vi "Radau5_Timestep Check.vi"(0 "time step":dbl, 5 "Initial time step":dbl, 7 "Max time step":dbl, 9 "Min time step":dbl, 11 "error in (no error)":errorcluster) -> (15 "error out":errorcluster)   [LabVIEW 2020, in "NI_DAE.lvlib"]
uses:
  <vilib>/gmath/NI_DAE.lvlib
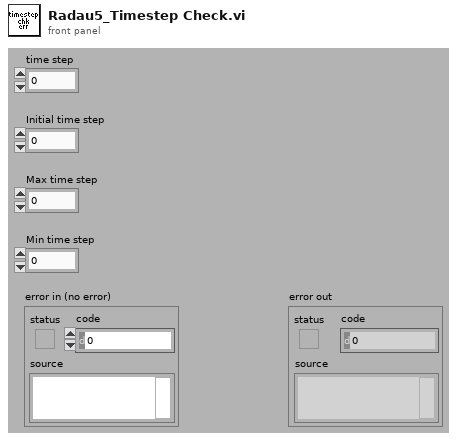
[diagram p1: front panel]
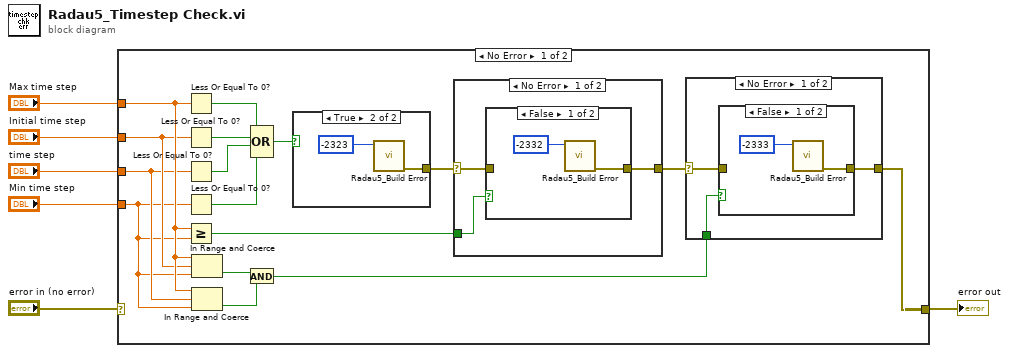
[diagram p0: block diagram]
diagram:
  n1 = case shown="No Error" "error in (no error)" {
    selector: "error in (no error)" -> [_ w39]
    tunnel: [w15 w39] -> w5
    tunnel: "time step" -> [w12 _]
    tunnel: "Initial time step" -> [w13 _]
    tunnel: "Max time step" -> [w14 _]
    tunnel: "Min time step" -> [w11 _]
    frame No Error {
      n2 = Less Or Equal To 0?(x=w14) -> (x <= 0?=w7:bool)
      n3 = Less Or Equal To 0?(x=w13) -> (x <= 0?=w8:bool)
      n4 = Less Or Equal To 0?(x=w12) -> (x <= 0?=w9:bool)
      n5 = Less Or Equal To 0?(x=w11) -> (x <= 0?=w10:bool)
      n6 = Greater Or Equal?(x=w14, y=w11) -> (x >= y?=w20:bool)
      n7 = In Range and Coerce(upper limit=w14, x=w13, lower limit=w11) -> (In Range?=w18:bool)  [unwired: 1 out]
      n8 = In Range and Coerce(upper limit=w14, x=w12, lower limit=w11) -> (In Range?=w17:bool)  [unwired: 1 out]
      n9 = And(x=w18, y=w17) -> (x .and. y?=w16:bool)
      n10 = Compound Arithmetic op=OR(w7, w8, w9, w10) -> (w22:bool)
      n11 = case shown="True" w22 {
        tunnel: [_ w38] -> w21
        frame False {
        }
        frame True {
          n12 = call <vilib>:"Radau5_Build Error.vi"("error code"=-2323 ("error.code")) -> ("error out"=w38:errorcluster)  [unwired: 10 in]
        }
      }
      n13 = case shown="No Error" w21 {
        selector: w21 -> [w30 w36]
        tunnel: w20 -> [w32 _]
        tunnel: [w31 w36] -> w19
        frame No Error {
          n14 = case shown="False" w32 {
            tunnel: [w33 w35] -> w31
            tunnel: w30 -> [_ w35]
            frame False {
              n15 = call <vilib>:"Radau5_Build Error.vi"("error code"=-2332 ("error.code")) -> ("error out"=w33:errorcluster)  [unwired: 10 in]
            }
            frame True {
            }
          }
        }
        frame Error {
        }
      }
      n16 = case shown="No Error" w19 {
        selector: w19 -> [w23 w29]
        tunnel: w16 -> [w25 _]
        tunnel: [w24 w29] -> w15
        frame No Error {
          n17 = case shown="False" w25 {
            tunnel: [w26 w28] -> w24
            tunnel: w23 -> [_ w28]
            frame False {
              n18 = call <vilib>:"Radau5_Build Error.vi"("error code"=-2333 ("error.code")) -> ("error out"=w26:errorcluster)  [unwired: 10 in]
            }
            frame True {
            }
          }
        }
        frame Error {
        }
      }
    }
    frame Error {
    }
  }
  "error out" <- w5
